vi "Autonomous Independent.vi"() -> ()   [LabVIEW 2013]
doc: "This VI is called when autonomous begins, and will automatically be terminated when autonomous ends. You can carry out timed or sensor driven robot movement independently without needing to return to the caller."
uses:
  <vilib>/Rock Robotics/WPI/Solenoid/WPI_SolenoidValue.ctl
  <vilib>/Rock Robotics/WPI/Relay/WPI_RelayValue.ctl
  Robot Global Data.vi
  <vilib>/Rock Robotics/WPI/Solenoid/WPI_SolenoidSetEnum.vi
  <vilib>/Rock Robotics/WPI/RobotDrive/WPI_RobotDriveArcadeDrive_Standard(NoSaturation).vi
  <vilib>/Rock Robotics/WPI/RobotDrive/WPI_RobotDriveGetSetRefNum.vi
  <vilib>/Rock Robotics/WPI/Joystick/WPI_JoystickGetSetRefNum.vi
  <vilib>/addons/control/pid/NI_PID_pid.lvlib
  <vilib>/addons/control/pid/pid.llb/PID (DBL).vi
  TargetType.ctl
panel:
  in  "Dist to drive":dbl=10000.0
  out "Go now or wait?":enum16{"Go Now", "Wait"}(ring)
  out "Stop Time":u32=1000
  in  "stop":bool
  out "Drive Forward Time":u32=1000
  out "Shoot Time":u32=1000
  out "Right? (T)":bool
  out "Position":T1
  in  "Launcher State":enum16{"Shoot", "Out", "Retract"}(ring)
  in  "Shooter Extended Time":u32=500
  out "Shooter Tick":u32
  out "Check Target Time":u32=5000
  out "Left?":bool
  out "Raise Arms Time":u32=1500
  in  "Up Position":dbl format="%.2f"
  out "Close Arms Time":u32=250
  out "Lower Arms Time":u32=1500
  in  "Down Position":dbl format="%.2f"
  out "Open Arms Time":u32=250
  in  "Auton State":T2(ring)
  out "Tick at start of Auton":u32
  out "Current Movement, for debugging":T3 {"Y Joystick Value" scale=1.0..-1.0; "X Joystick Value" scale=-1.0..1.0}
  in  "Array of robot movements":T4(array[cluster]) {"Y Joystick Value" scale=1.0..-1.0; "X Joystick Value" scale=-1.0..1.0}
  # "Be sure to right-click and choose Data Operations>>Make Current Value default if you want to save the array values with the VI"
  # "Main State Machine"
  # "Shooter State Machine"
  # "Disabled"
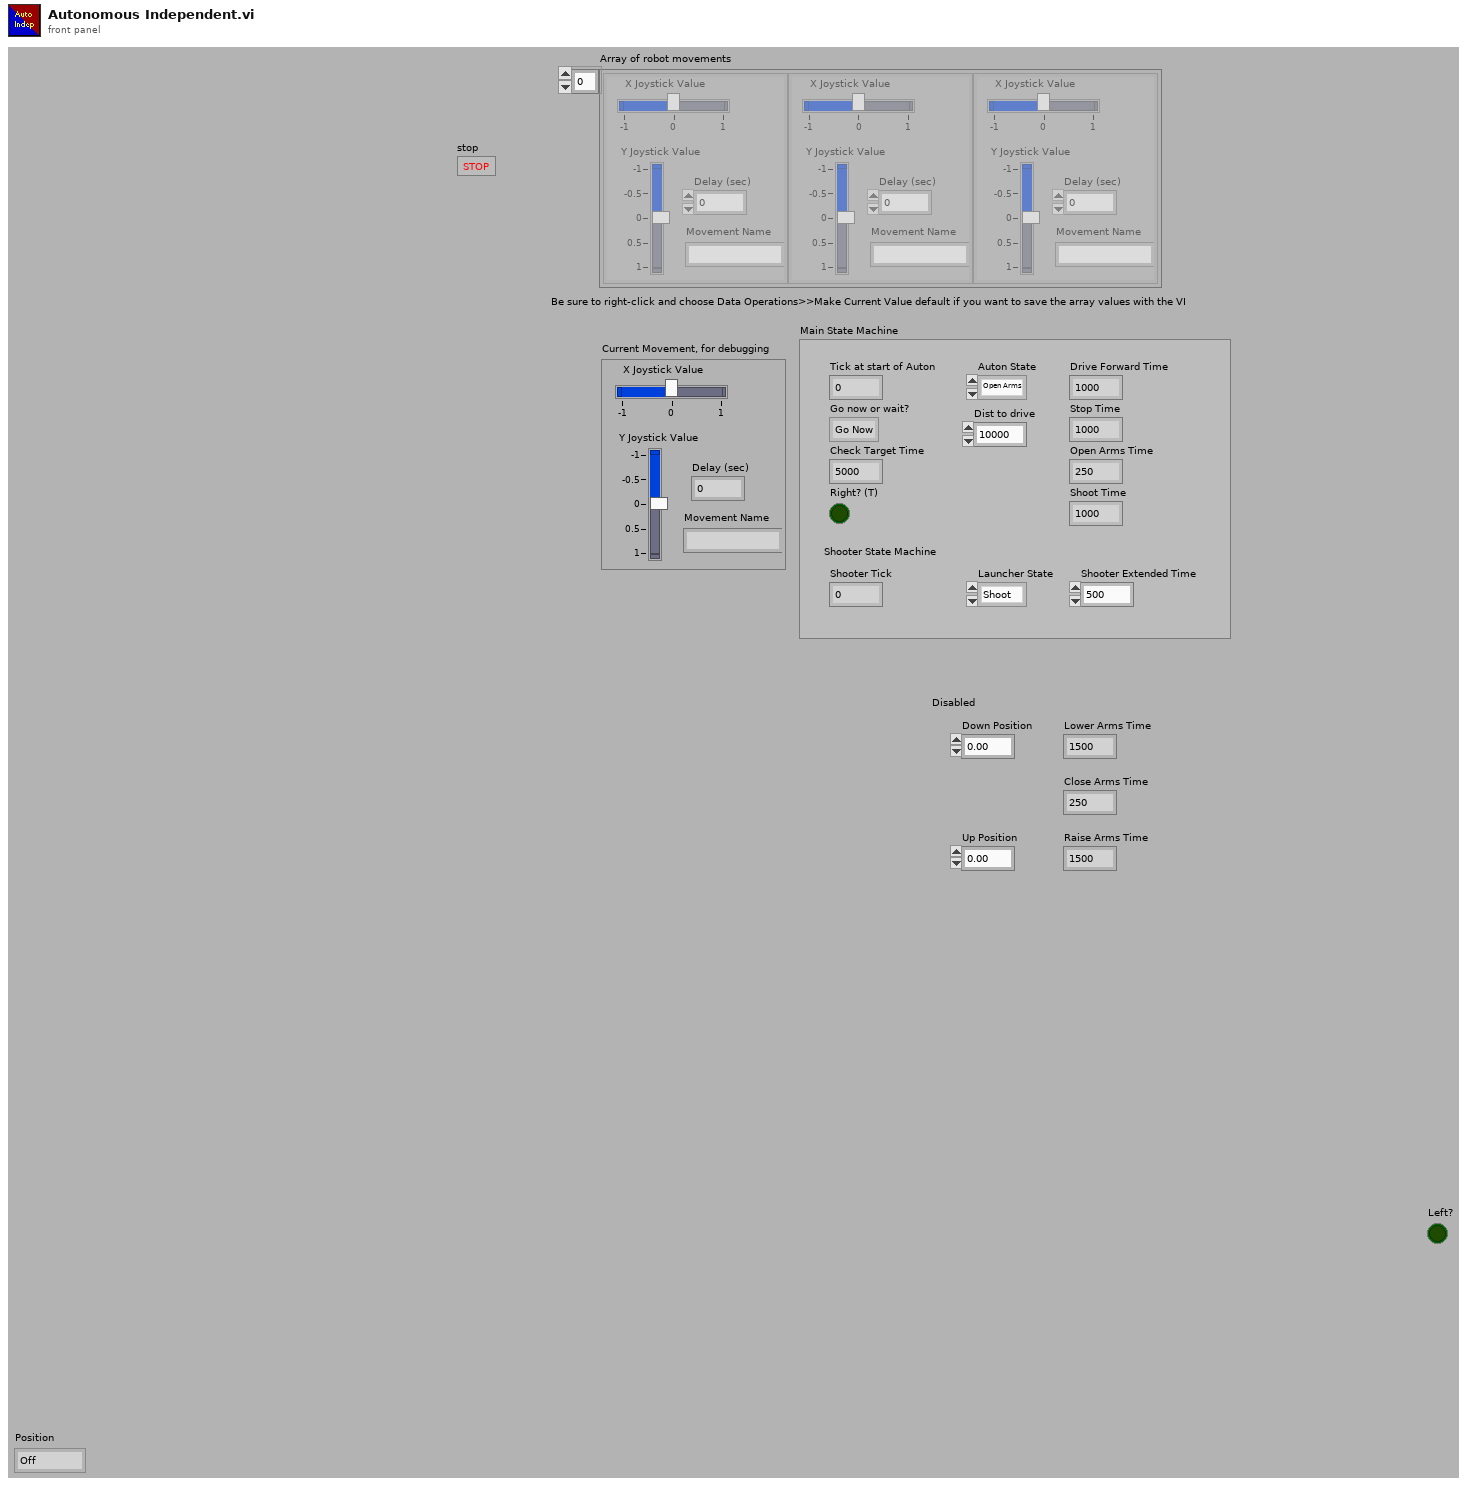
[diagram p1: front panel]
types:
  T1 = typedef "WPI_SolenoidValue.ctl" = enum16{"Off", "On", "Forward", "Reverse"}
  T2 = enum16{"Open Arms", "Lower Arms", "Close Arms", "Raise Arms", "Check Target", "Shoot", "Drive Forward", "Stop"}
  T3 = cluster{"X Joystick Value":dbl, "Y Joystick Value":dbl, "Delay (sec)":dbl, "Movement Name":string}
  T4 = cluster{"X Joystick Value":dbl, "Y Joystick Value":dbl, "Delay (sec)":dbl, "Movement Name":string}[]
  T5 = typedef "WPI_JoystickDevRef.ctl" = cluster{"Device":T6}
  T6 = typedef "WPI_JoystickDeviceEnum.ctl" = enum16{"USB 1", "USB 2", "USB 3", "USB 4", "Kinect 1", "Kinect 2"}
  T7 = cluster{"axis 1 (x)":dbl, "axis 2 (y)":dbl, "axis 3 (throttle)":dbl, "axis 4":dbl, "axis 5":dbl, "axis 6":dbl}
  T8 = typedef "WPI_RelayValue.ctl" = enum16{"Off", "On", "Forward", "Reverse"}
  T9 = typedef "TargetType.ctl" = enum16{"Not Hot", "Hot"}
  T10 = enum16{"Open Arms", "Lower Arms", "Close Arms", "Raise Arms", "Check Target", "Shoot", "Drive Forward"}
  T11 = cluster{"proportional gain (Kc)":dbl, "integral time (Ti, min)":dbl, "derivative time (Td, min)":dbl}
  T12 = typedef "WPI_SolenoidDevRef.ctl" = cluster{"DevStatus":errorcluster, "Solenoid Module":T13, "Forward Solenoid Channel":T14, "Reverse Solenoid Channel":T14}
  T13 = typedef "FPGA_TypedefSolenoidModule.ctl" = enum16{"Solenoid Module 1", "Solenoid Module 2"}
  T14 = typedef "WPI_SolenoidChannel.ctl" = enum8{"Solenoid 1", "Solenoid 2", "Solenoid 3", "Solenoid 4", "Solenoid 5", "Solenoid 6", "Solenoid 7", "Solenoid 8", "Invalid"}
  T15 = typedef "WPI_RelayDevRef.ctl" = cluster{"DevStatus":errorcluster, "Relay Channel":T16, "Digital Module":T17, "Relay Direction":T18}
  T16 = typedef "FPGA_DIORelayChannel.ctl" = enum8{"Relay 1", "Relay 2", "Relay 3", "Relay 4", "Relay 5", "Relay 6", "Relay 7", "Relay 8", "Invalid"}
  T17 = typedef "FPGA_TypedefDigitalModule.ctl" = enum16{"Digital Module 1", "Digital Module 2"}
  T18 = typedef "WPI_RelayDirection.ctl" = enum16{"Both directions", "Forward only", "Reverse only"}
  T19 = cluster{"Distance (ft)":dbl, "Target Center (-1 to 1)":cluster{"X":dbl, "Y":dbl}, "Left":bool, "State":T9}
  T20 = typedef "WPI_RobotDriveDevRef.ctl" = cluster{"DevStatus":errorcluster, "Motors[]":T21[], "Square Inputs":bool, "Max Output":dbl, "Isochronous":bool}
  T21 = typedef "WPI_MotorControlDeviceRef.ctl" = cluster{"DeviceStatus":errorcluster, "Type":enum16{"PWM", "CAN"}, "PWM":cluster{"Digital Module":T17, "PWM Channel":T22, "DeadBand":T23}, "CAN":cluster{"Device Number":u8, "Control Mode":T24, "Semaphore":T25, "Max Vout":dbl}, "Invert":bool, "TransformRef":T26, "InvTransformRef":T26}
  T22 = typedef "FPGA_DIOPWMChannel.ctl" = enum8{"PWM 1", "PWM 2", "PWM 3", "PWM 4", "PWM 5", "PWM 6", "PWM 7", "PWM 8", "PWM 9", "PWM 10", "Invalid"}
  T23 = typedef "WPI_PWMDeadband.ctl" = cluster{"Name":string, "maxPositivePwm":i32, "minPositivePwm":i32, "centerPwm":i32, "maxNegativePwm":i32, "minNegativePwm":i32, "angularRange":u16}
  T24 = typedef "WPI_CANJaguar_ControlMode.ctl" = enum8{"Percent VBus", "Current", "Speed", "Position", "Voltage"}
  T25 = typedef "Semaphore RefNum" = refnum<k1>
  T26 = typedef "WPI_PWMTransform_ConPane.ctl" = refnum<vi>
  T27 = typedef "WPI_AnalogChannelDevRef.ctl" = cluster{"DevStatus":errorcluster, "Analog Module":T28, "Analog Channel":T29}
  T28 = typedef "FPGA_TypedefAnalogModule.ctl" = enum16{"Analog Module 1", "Analog Module 2"}
  T29 = typedef "FPGA_AIChannel.ctl" = enum8{"AI 1", "AI 2", "AI 3", "AI 4", "AI 5", "AI 6", "AI 7", "AI 8", "Invalid"}
  T30 = typedef "WPI_EncoderDevRef.ctl" = cluster{"DevStatus":errorcluster, "EncoderIndex":T31, "CounterIndex":T32, "DistancePerCount":dbl, "Decoding Type":T33}
  T31 = typedef "FPGA_EncoderIdx.ctl" = enum8{"Enc 0", "Enc 1", "Enc 2", "Enc 3", "Invalid"}
  T32 = typedef "FPGA_CounterCtrSystemIndex.ctl" = enum8{"Ctr 0", "Ctr 1", "Ctr 2", "Ctr 3", "Ctr 4", "Ctr 5", "Ctr 6", "Ctr 7", "Invalid"}
  T33 = typedef "WPI_EncoderType.ctl" = enum16{"1x", "2x", "4x"}
  T34 = enum16{"Target Right", "No Target", "Target Left"}
  T35 = typedef "WPI_DigitalInputDevRef.ctl" = cluster{"DevStatus":errorcluster, "DIO Channel":T36, "Digital Module":T17}
  T36 = typedef "FPGA_DIOChannel.ctl" = enum8{"DIO 1", "DIO 2", "DIO 3", "DIO 4", "DIO 5", "DIO 6", "DIO 7", "DIO 8", "DIO 9", "DIO 10", "DIO 11", "DIO 12", "DIO 13", "DIO 14", "Invalid"}
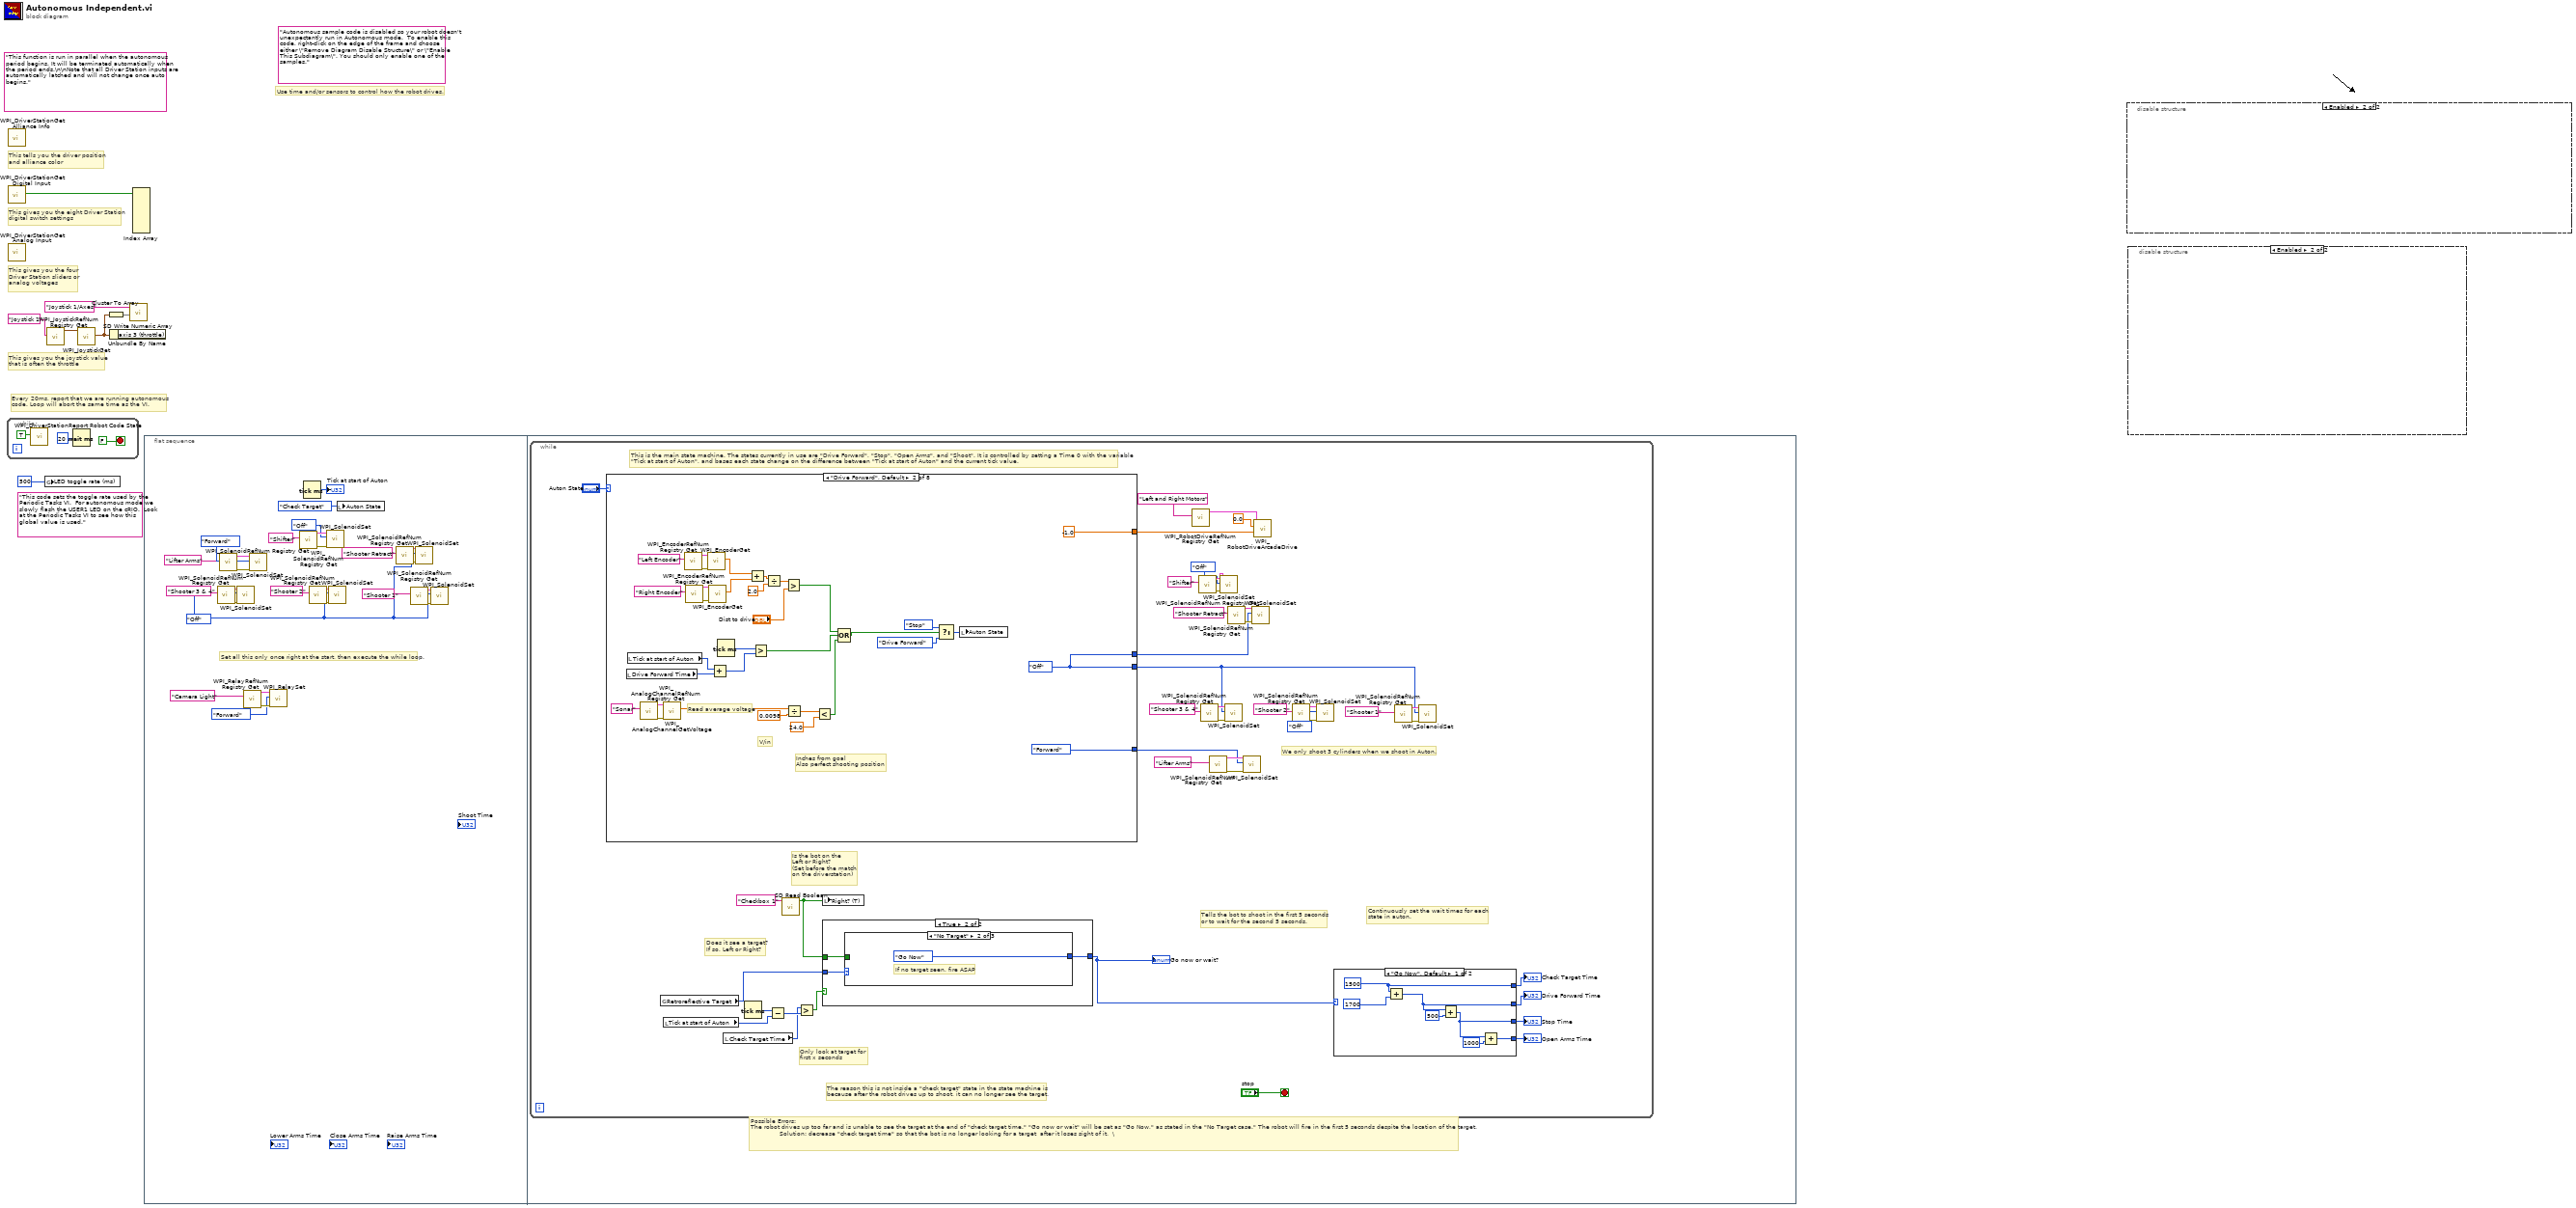
[diagram p0: block diagram]
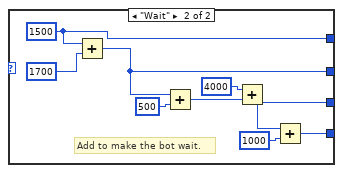
[diagram p2: hidden frame]
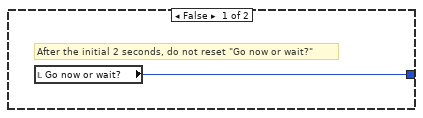
[diagram p3: hidden frame]
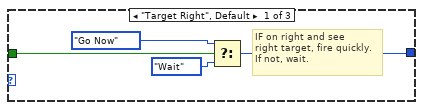
[diagram p4: hidden frame]
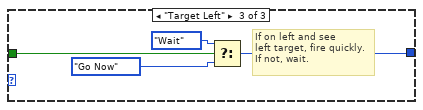
[diagram p5: hidden frame]
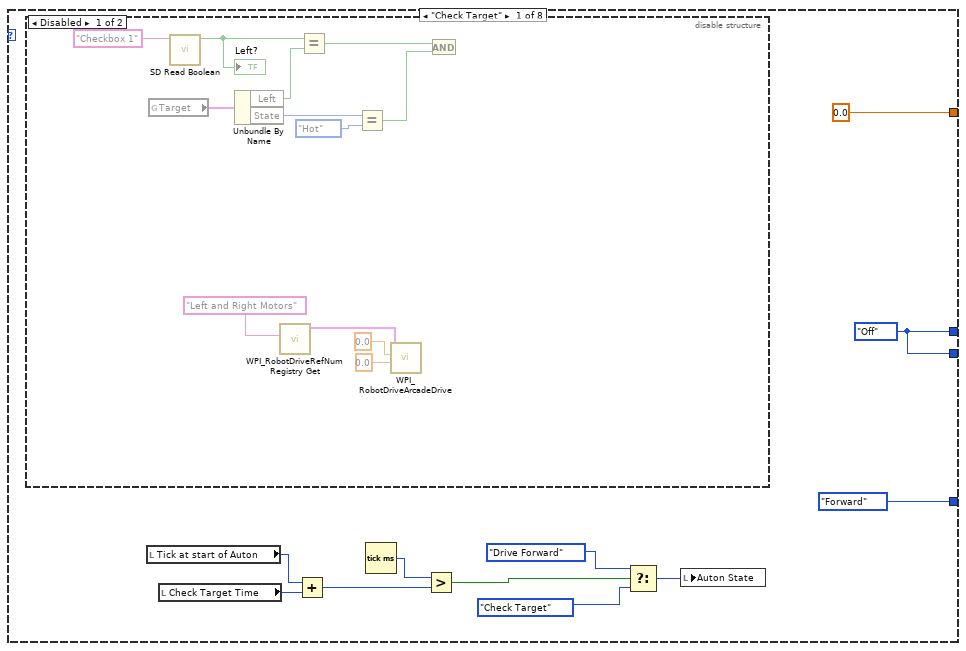
[diagram p6: hidden frame]
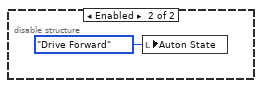
[diagram p7: hidden frame]
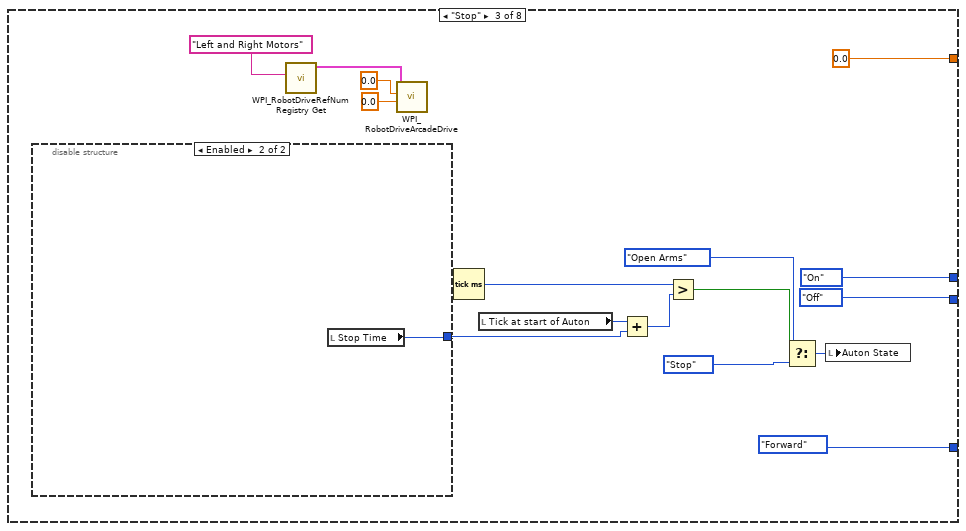
[diagram p8: hidden frame]
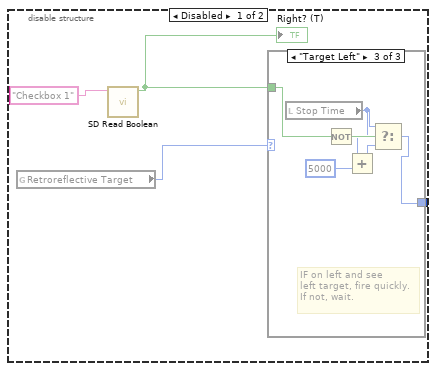
[diagram p9: hidden frame]
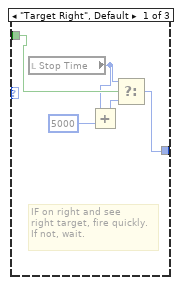
[diagram p10: hidden frame]
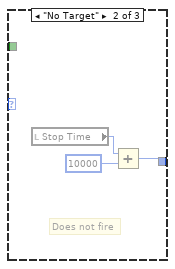
[diagram p11: hidden frame]
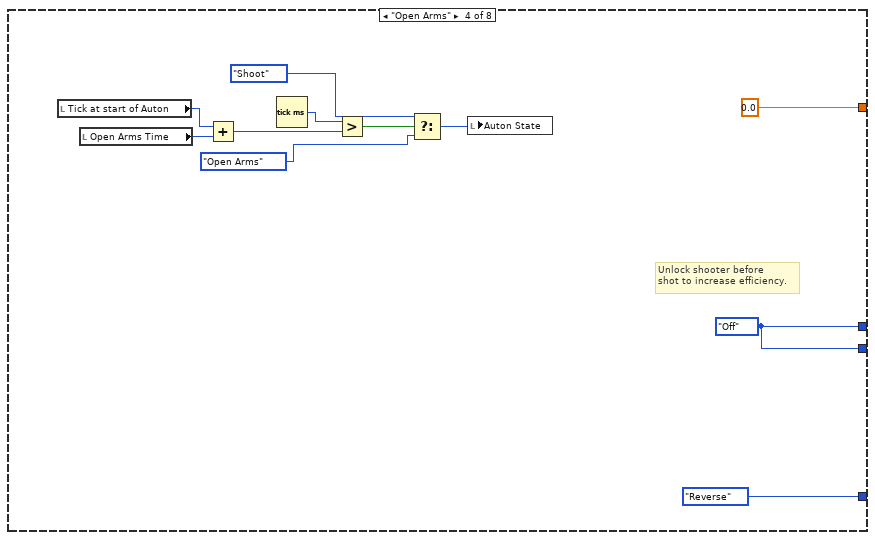
[diagram p12: hidden frame]
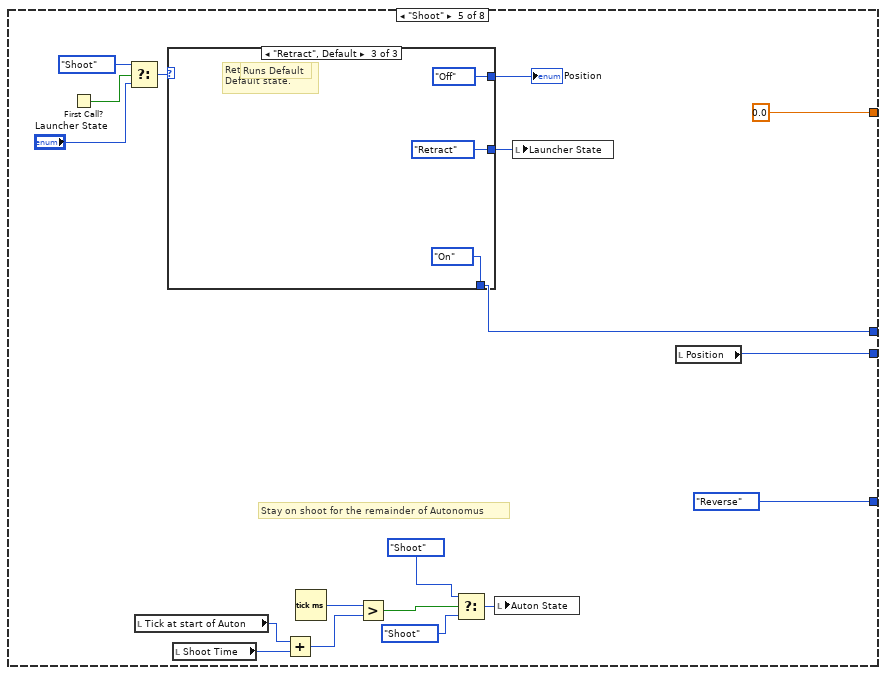
[diagram p13: hidden frame]
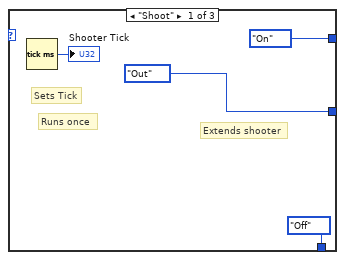
[diagram p14: hidden frame]
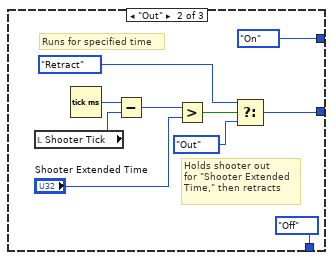
[diagram p15: hidden frame]
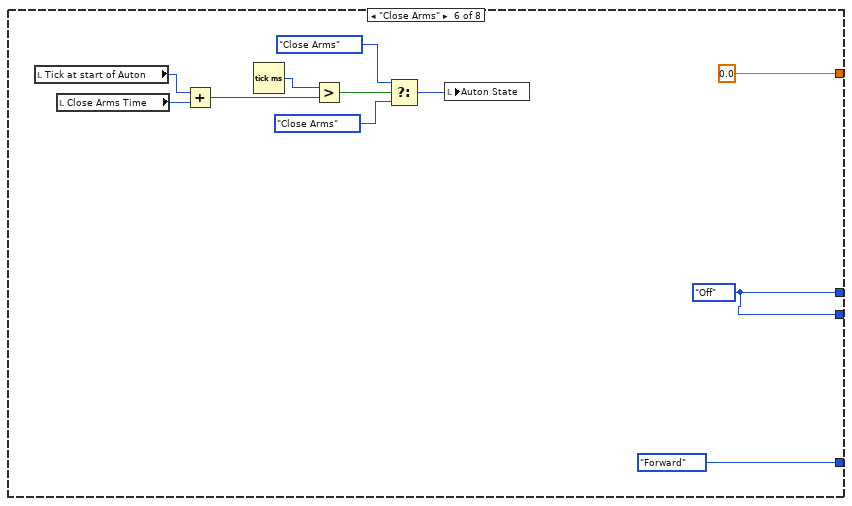
[diagram p16: hidden frame]
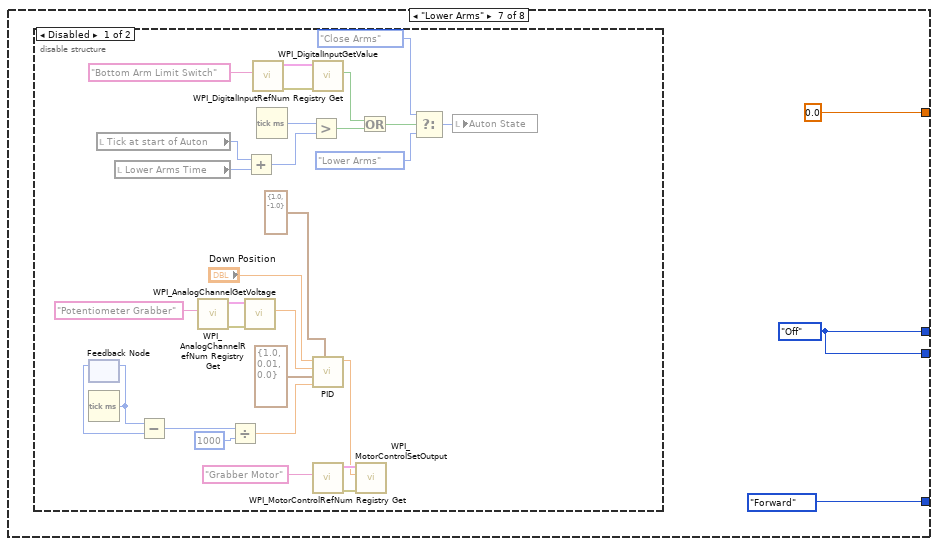
[diagram p17: hidden frame]
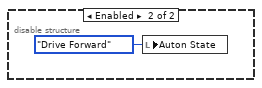
[diagram p18: hidden frame]
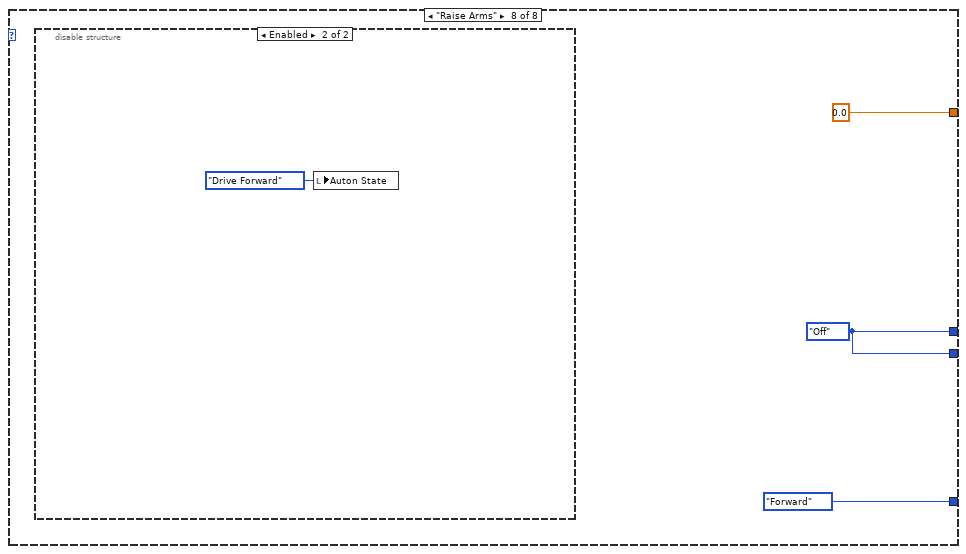
[diagram p19: hidden frame]
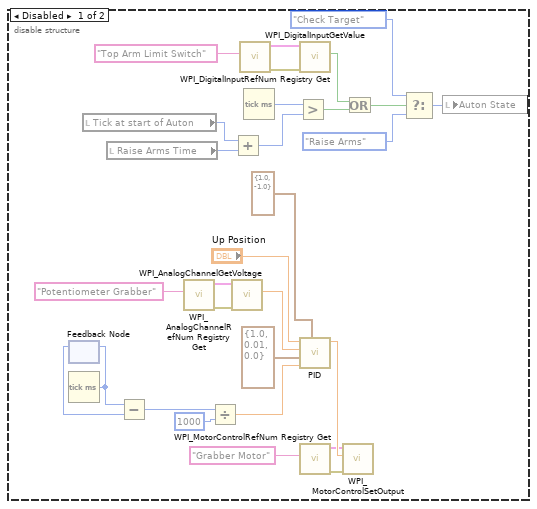
[diagram p20: hidden frame]
diagram:
  (unwired) "This code sets the toggle rate used by the Periodic Tasks VI.  For autonomous mode we slowly flash the USER1 LED on the cRIO.  Look at the Periodic Tasks VI to see how this global value is used."
  (unwired) "Autonomous sample code is disabled so your robot doesn't unexpectantly run in Autonomous mode.  To enable this code, right-click on the edge of the frame and choose either \"Remove Diagram Disable Structure\" or \"Enable This Subdiagram\". You should only enable one of the samples."
  (unwired) "This function is run in parallel when the autonomous period begins. It will be terminated automatically when the period ends.\n\nNote that all Driver Station inputs are automatically latched and will not change once auto begins."
  # "Every 20ms, report that we are running autonomous\ncode. Loop will abort the same time as the VI."
  # "This gives you the joystick value\nthat is often the throttle"
  # "Use time and/or sensors to control how the robot drives."
  # "This tells you the driver position\nand alliance color"
  # "This gives you the eight Driver Station\ndigital switch settings"
  # "This gives you the four\nDriver Station sliders or\nanalog voltages"
  n1 = while {
    stop <- FALSE stop-if-true
    n2 = call <vilib>:"WPI_DriverStationReport Robot Code State.vi"("Autonomous"=TRUE) -> ()  [unwired: 10 in, 1 out]
    n3 = Wait (ms)(milliseconds to wait=u32 20) -> ()  [unwired: 1 out]
  }
  n4 = call <vilib>:"WPI_DriverStationGet Alliance Info.vi"() -> ()  [unwired: 12 out]
  n5 = call <vilib>:"WPI_DriverStationGet Digital Input.vi"() -> ("Driver Station Digital Input (1-8)"=w7:bool[])  [unwired: 11 out]
  n6 = call <vilib>:"WPI_DriverStationGet Analog Input.vi"() -> ()  [unwired: 12 out]
  n7 = global write "Robot Global Data.vi" "LED toggle rate (ms)"(u32 500 ("LED ms toggle rate")) -> ()
  n8 = call <vilib>:"WPI_JoystickRefNum Registry Get.vi"("refnum name"="Joystick 1") -> ("JoystickDevRef"=w5:T5)  [unwired: 1 in, 9 out]
  n9 = call <vilib>:"WPI_JoystickGet.vi"("JoystickDevRef"=w5) -> ("Axes"=w2:T7)  [unwired: 1 in, 5 out]
  n10 = Cluster To Array(cluster=w2) -> (array=w3:dbl[])
  n11 = Unbundle By Name(w2) -> ()  [unwired: 1 out]
  n12 = call <vilib>:"SD Write Numeric Array.vi"("Numeric Array"=w3, "Name"="Joystick 1/Axes") -> ()  [unwired: 8 in, 2 out]
  n13 = Index Array(array=w7) -> ()  [unwired: 8 in, 8 out]
  n14 = flat-sequence {
    frame #0 {
      w23 = WPI_SolenoidValue."Off" ("x")
      # "Set all this only once right at the start, then execute the while loop."
      n15 = call <vilib>:"WPI_SolenoidRefNum Registry Get.vi"("refnum name"="Shooter 3 & 4") -> ("error out"=w30:errorcluster, "SolenoidDevRef"=w34:T12)  [unwired: 9 in]
      n16 = call <vilib>:"WPI_SolenoidRefNum Registry Get.vi"("refnum name"="Lifter Arms") -> ("error out"=w17:errorcluster, "SolenoidDevRef"=w18:T12)  [unwired: 9 in]
      n17 = call-poly <vilib>:"WPI_SolenoidSet.vi"("error in (no error)"=w30, "Value"=w23, "SolenoidDevRef"=w34) -> ()  [unwired: 7 in, 2 out]
      n18 = call <vilib>:"WPI_RelayRefNum Registry Get.vi"("refnum name"="Camera Light") -> ("error out"=w14:errorcluster, "RelayDevRef"=w13:T15)  [unwired: 9 in]
      n19 = call-poly <vilib>:"WPI_SolenoidSet.vi"("error in (no error)"=w17, "Value"=WPI_SolenoidValue."Forward", "SolenoidDevRef"=w18) -> ()  [unwired: 7 in, 2 out]
      n20 = call <vilib>:"WPI_RelaySet.vi"("error in (no error)"=w14, "RelayValue"=WPI_RelayValue."Forward", "RelayDevRef"=w13) -> ()  [unwired: 7 in, 2 out]
      n21 = call <vilib>:"WPI_SolenoidRefNum Registry Get.vi"("refnum name"="Shifter") -> ("error out"=w21:errorcluster, "SolenoidDevRef"=w20:T12)  [unwired: 9 in]
      n22 = Tick Count (ms)() -> (millisecond timer value=→"Tick at start of Auton":u32)
      n23 = call <vilib>:"WPI_SolenoidRefNum Registry Get.vi"("refnum name"="Shooter 2") -> ("error out"=w27:errorcluster, "SolenoidDevRef"=w35:T12)  [unwired: 9 in]
      n24 = call-poly <vilib>:"WPI_SolenoidSet.vi"("error in (no error)"=w21, "Value"=WPI_SolenoidValue."Off", "SolenoidDevRef"=w20) -> ()  [unwired: 7 in, 2 out]
      n25 = call-poly <vilib>:"WPI_SolenoidSet.vi"("error in (no error)"=w27, "Value"=w23, "SolenoidDevRef"=w35) -> ()  [unwired: 7 in, 2 out]
      n26 = local write "Auton State"(T2."Check Target" ("Auton State")) -> ()
      n27 = call <vilib>:"WPI_SolenoidRefNum Registry Get.vi"("refnum name"="Shooter Retract") -> ("error out"=w25:errorcluster, "SolenoidDevRef"=w24:T12)  [unwired: 9 in]
      n28 = call <vilib>:"WPI_SolenoidRefNum Registry Get.vi"("refnum name"="Shooter 1") -> ("error out"=w32:errorcluster, "SolenoidDevRef"=w33:T12)  [unwired: 9 in]
      n29 = call-poly <vilib>:"WPI_SolenoidSet.vi"("error in (no error)"=w25, "Value"=w23, "SolenoidDevRef"=w24) -> ()  [unwired: 7 in, 2 out]
      n30 = call-poly <vilib>:"WPI_SolenoidSet.vi"("error in (no error)"=w32, "Value"=w23, "SolenoidDevRef"=w33) -> ()  [unwired: 7 in, 2 out]
    }
    frame #1 {
      # "Possible Errors:\nThe robot drives up too far and is unable to see the target at the end of \"check target time.\" \"Go now or wait\" will be set as \"Go Now,\" as stated in the \"No Target case.\" The robot will fire in the first 5 seconds despite the location of the target.\n               Solution: decrease \"check target time\" so that the bot is no longer looking for a target  after it loses sight of it.  \\"
      n31 = while {
        stop <- "stop" stop-if-true
        # "We only shoot 3 cylinders when we shoot in Auton."
        # "This is the main state machine. The states currently in use are \"Drive Forward\", \"Stop\", \"Open Arms\", and \"Shoot\". It is controlled by setting a Time 0 with the variable\n\"Tick at start of Auton\", and bases each state change on the difference between \"Tick at start of Auton\" and the current tick value."
        # "The reason this is not inside a \"check target\" state in the state machine is \nbecause after the robot drives up to shoot, it can no longer see the target."
        # "Continuously set the wait times for each\nstate in auton."
        # "Tells the bot to shoot in the first 5 seconds\nor to wait for the second 5 seconds."
        # "Is the bot on the\nLeft or Right?\n(Set before the match\non the driverstation)"
        # "Does it see a target?\nIf so, Left or Right?"
        # "Only look at target for \nfirst x seconds"
        n32 = case shown="\"Drive Forward\", Default" "Auton State" {
          tunnel: [w117 w159 WPI_SolenoidValue."Off" ("x") w204 w216 w252 w261 w294] -> w65
          tunnel: [w117 w159 WPI_SolenoidValue."On" ("x") w204 w213 w252 w261 w294] -> w64
          tunnel: [0.0 ("Y axis value") -1.0 ("Y axis value") 0.0 ("Y axis value") 0.0 ("Y axis value") 0.0 ("Y axis value") 0.0 ("Y axis value") 0.0 ("Y axis value") 0.0 ("Y axis value")] -> w60
          tunnel: [WPI_SolenoidValue."Forward" ("Value") WPI_SolenoidValue."Forward" ("Value") WPI_SolenoidValue."Forward" ("Value") WPI_SolenoidValue."Reverse" ("Value") WPI_SolenoidValue."Reverse" ("Value") WPI_SolenoidValue."Forward" ("Value") WPI_SolenoidValue."Forward" ("Value") WPI_SolenoidValue."Forward" ("Value")] -> w52
          frame "Check Target" {
            w117 = WPI_SolenoidValue."Off" ("x")
            n33 = disable-structure shown="Disabled" {
              frame Disabled {
                n34 = global read "Robot Global Data.vi" "Target"() -> (w132:T19)
                n35 = call <vilib>:"SD Read Boolean.vi"("Name"="Checkbox 1" ("refnum name")) -> ("Boolean"=w127:bool)  [unwired: 8 in, 2 out]
                "Left?" <- w127
                n36 = Unbundle By Name(w132) -> ("Left"=w128:bool, "State"=w131:T9)
                n37 = call <vilib>:"WPI_RobotDriveRefNum Registry Get.vi"("refnum name"="Left and Right Motors") -> ("RobotDriveDevRef"=w120:T20)  [unwired: 1 in, 9 out]
                n38 = Equal?(x=w127, y=w128) -> (x = y?=w125:bool)
                n39 = Equal?(x=w131, y=TargetType."Hot") -> (x = y?=w126:bool)
                n40 = call-poly <vilib>:"WPI_RobotDriveArcadeDrive.vi"("Y axis value"=0.0, "X axis value"=0.0, "RobotDriveDevRef"=w120) -> ()  [unwired: 6 in, 3 out]
                n41 = And(x=w125, y=w126) -> (x .and. y?=w124:bool)
              }
              frame Enabled {
                n42 = local write "Auton State"(T2."Drive Forward" ("Auton State")) -> ()
              }
            }
            n43 = local read "Tick at start of Auton"() -> (w113:u32)
            n44 = local read "Check Target Time"() -> (w111:u32)
            n45 = Add(x=w113, y=w111) -> (x+y=w112:u32)
            n46 = Tick Count (ms)() -> (millisecond timer value=w114:u32)
            n47 = Greater?(x=w114, y=w112) -> (0:w109:bool)
            n48 = Select(t=T2."Drive Forward" ("Auton State"), s=w109, f=T2."Check Target" ("Auton State")) -> (s? t:f=w115:T2)
            n49 = local write "Auton State"(w115) -> ()
          }
          frame "Drive Forward", Default {
            w159 = WPI_SolenoidValue."Off" ("Value")
            # "Inches from goal\nAlso perfect shooting position"
            # "V/in"
            # "Read average voltage"
            n50 = local read "Drive Forward Time"() -> (w166:u32)
            n51 = local read "Tick at start of Auton"() -> (w164:u32)
            n52 = call <vilib>:"WPI_AnalogChannelRefNum Registry Get.vi"("refnum name"="Sonar") -> ("error out"=w143:errorcluster, "AIDeviceRef"=w138:T27)  [unwired: 9 in]
            n53 = call <vilib>:"WPI_AnalogChannelGetVoltage.vi"("error in (no error)"=w143, "AIDeviceRef"=w138) -> ("Voltage"=w144:dbl)  [unwired: 7 in, 2 out]
            n54 = call <vilib>:"WPI_EncoderRefNum Registry Get.vi"("refnum name"="Left Encoder") -> ("error out"=w156:errorcluster, "EncoderDevRef"=w155:T30)  [unwired: 9 in]
            n55 = call <vilib>:"WPI_EncoderRefNum Registry Get.vi"("refnum name"="Right Encoder") -> ("error out"=w151:errorcluster, "EncoderDevRef"=w152:T30)  [unwired: 9 in]
            n56 = call <vilib>:"WPI_EncoderGet.vi"("error in (no error)"=w156, "EncoderDevRef"=w155) -> ("Distance"=w150:dbl)  [unwired: 4 in, 5 out]
            n57 = call <vilib>:"WPI_EncoderGet.vi"("error in (no error)"=w151, "EncoderDevRef"=w152) -> ("Distance"=w149:dbl)  [unwired: 4 in, 5 out]
            n58 = Add(x=w164, y=w166) -> (x+y=w165:u32)
            n59 = Tick Count (ms)() -> (millisecond timer value=w163:u32)
            n60 = Add(x=w150, y=w149) -> (x+y=w148:dbl)
            n61 = Greater?(x=w163, y=w165) -> (0:w135:bool)
            n62 = Divide(x=w148, y=2.0) -> (x/y=w146:dbl)
            n63 = Greater?(x=w146, y="Dist to drive") -> (0:w136:bool)
            n64 = Divide(x=w144, y=0.0098) -> (x/y=w140:dbl)
            n65 = Less?(x=w140, y=24.0) -> (x < y?=w134:bool)
            n66 = Compound Arithmetic op=OR(w136, w135, w134) -> (w137:bool)
            n67 = Select(t=T2."Stop" ("Auton State"), s=w137, f=T2."Drive Forward" ("Auton State")) -> (s? t:f=w162:T2)
            n68 = local write "Auton State"(w162) -> ()
          }
          frame "Stop" {
            n69 = disable-structure shown="Enabled" {
              disable-tunnel: [w183 w201] -> w167
              frame Disabled {
                n70 = global read "Robot Global Data.vi" "Retroreflective Target"() -> (w185:T34)
                n71 = call <vilib>:"SD Read Boolean.vi"("Name"="Checkbox 1" ("refnum name")) -> ("Boolean"=w184:bool)  [unwired: 8 in, 2 out]
                "Right? (T)" <- w184
                n72 = case shown="\"Target Left\"" w185 {
                  tunnel: w184 -> [w188 _ w200]
                  tunnel: [w189 w194 w195] -> w183
                  frame "Target Right", Default {
                    # "IF on right and see\nright target, fire quickly.\nIf not, wait."
                    n73 = local read "Stop Time"() -> (w187:u32)
                    n74 = Add(x=w187, y=u32 5000) -> (x+y=w191:u32)
                    n75 = Select(t=w187, s=w188, f=w191) -> (s? t:f=w189:u32)
                  }
                  frame "No Target" {
                    # "Does not fire"
                    n76 = local read "Stop Time"() -> (w193:u32)
                    n77 = Add(x=w193, y=u32 10000) -> (x+y=w194:u32)
                  }
                  frame "Target Left" {
                    # "IF on left and see\nleft target, fire quickly.\nIf not, wait."
                    n78 = local read "Stop Time"() -> (w198:u32)
                    n79 = Not(x=w200) -> (.not. x?=w199:bool)
                    n80 = Add(x=w198, y=u32 5000) -> (x+y=w197:u32)
                    n81 = Select(t=w198, s=w199, f=w197) -> (s? t:f=w195:u32)
                  }
                }
              }
              frame Enabled {
                n82 = local read "Stop Time"() -> (w201:u32)
              }
            }
            n83 = call <vilib>:"WPI_RobotDriveRefNum Registry Get.vi"("refnum name"="Left and Right Motors") -> ("RobotDriveDevRef"=w179:T20)  [unwired: 1 in, 9 out]
            n84 = call-poly <vilib>:"WPI_RobotDriveArcadeDrive.vi"("Y axis value"=0.0, "X axis value"=0.0, "RobotDriveDevRef"=w179) -> ()  [unwired: 6 in, 3 out]
            n85 = Tick Count (ms)() -> (millisecond timer value=w173:u32)
            n86 = local read "Tick at start of Auton"() -> (w174:u32)
            n87 = Add(x=w174, y=w167) -> (x+y=w175:u32)
            n88 = Greater?(x=w173, y=w175) -> (0:w171:bool)
            n89 = Select(t=T2."Open Arms" ("Auton State"), s=w171, f=T2."Stop" ("Auton State")) -> (s? t:f=w172:T2)
            n90 = local write "Auton State"(w172) -> ()
          }
          frame "Open Arms" {
            w204 = WPI_SolenoidValue."Off" ("Value")
            # "Unlock shooter before\nshot to increase efficiency."
            n91 = local read "Tick at start of Auton"() -> (w211:u32)
            n92 = local read "Open Arms Time"() -> (w208:u32)
            n93 = Add(x=w211, y=w208) -> (x+y=w210:u32)
            n94 = Tick Count (ms)() -> (millisecond timer value=w212:u32)
            n95 = Greater?(x=w212, y=w210) -> (0:w209:bool)
            n96 = Select(t=T2."Shoot" ("Auton State"), s=w209, f=T2."Open Arms" ("Auton State")) -> (s? t:f=w205:T2)
            n97 = local write "Auton State"(w205) -> ()
          }
          frame "Shoot" {
            # "Stay on shoot for the remainder of Autonomus"
            n98 = First Call?() -> (First Call?: T/F=w225:bool)
            n99 = Select(t=enum16{"Shoot", "Out", "Retract"}."Shoot", s=w225, f="Launcher State") -> (s? t:f=w229:enum16{"Shoot", "Out", "Retract"})
            n100 = local read "Tick at start of Auton"() -> (w222:u32)
            n101 = case shown="\"Retract\", Default" w229 {
              tunnel: [WPI_SolenoidValue."On" ("Value") WPI_SolenoidValue."On" ("Value") WPI_SolenoidValue."Off" ("Value")] -> w226
              tunnel: [enum16{"Shoot", "Out", "Retract"}."Out" ("Launcher State") w237 enum16{"Shoot", "Out", "Retract"}."Retract" ("Launcher State")] -> w227
              tunnel: [WPI_SolenoidValue."Off" ("t") WPI_SolenoidValue."Off" ("t") WPI_SolenoidValue."On" ("t")] -> w213
              frame "Shoot" {
                # "Runs once"
                # "Sets Tick"
                # "Extends shooter"
                n102 = Tick Count (ms)() -> (millisecond timer value=→"Shooter Tick":u32)
              }
              frame "Out" {
                # "Runs for specified time"
                # "Holds shooter out\nfor \"Shooter Extended\nTime,\" then retracts"
                n103 = local read "Shooter Tick"() -> (w243:u32)
                n104 = Tick Count (ms)() -> (millisecond timer value=w244:u32)
                n105 = Subtract(x=w244, y=w243) -> (x-y=w242:u32)
                n106 = Greater?(x=w242, y="Shooter Extended Time") -> (0:w241:bool)
                n107 = Select(t=enum16{"Shoot", "Out", "Retract"}."Retract" ("Launcher State"), s=w241, f=enum16{"Shoot", "Out", "Retract"}."Out" ("Launcher State")) -> (s? t:f=w237:enum16{"Shoot", "Out", "Retract"})
              }
              frame "Retract", Default {
                # "Runs Default"
                # "Retracts Shooter, \nDefault state."
              }
            }
            "Position" <- w226
            n108 = local read "Shoot Time"() -> (w224:u32)
            n109 = Add(x=w222, y=w224) -> (x+y=w223:u32)
            n110 = Tick Count (ms)() -> (millisecond timer value=w221:u32)
            n111 = Greater?(x=w221, y=w223) -> (0:w219:bool)
            n112 = Select(t=T2."Shoot" ("Auton State"), s=w219, f=T2."Shoot" ("Auton State")) -> (s? t:f=w220:T2)
            n113 = local write "Auton State"(w220) -> ()
            n114 = local write "Launcher State"(w227) -> ()
            n115 = local read "Position"() -> (w216:T1)
          }
          frame "Close Arms" {
            w252 = WPI_SolenoidValue."Off" ("x")
            n116 = local read "Tick at start of Auton"() -> (w255:u32)
            n117 = local read "Close Arms Time"() -> (w258:u32)
            n118 = Add(x=w255, y=w258) -> (x+y=w256:u32)
            n119 = Tick Count (ms)() -> (millisecond timer value=w254:u32)
            n120 = Greater?(x=w254, y=w256) -> (0:w257:bool)
            n121 = Select(t=T2."Close Arms" ("Auton State"), s=w257, f=T2."Close Arms" ("Auton State")) -> (s? t:f=w253:T2)
            n122 = local write "Auton State"(w253) -> ()
          }
          frame "Lower Arms" {
            w261 = WPI_SolenoidValue."Off" ("x")
            n123 = disable-structure shown="Disabled" {
              frame Disabled {
                n124 = feedback #1() -> (w285:u32)  [unwired: 1 in]
                n125 = Tick Count (ms)() -> (millisecond timer value=w286:u32)
                n126 = feedback-in #1(w286) -> ()
                n127 = local read "Tick at start of Auton"() -> (w267:u32)
                n128 = local read "Lower Arms Time"() -> (w265:u32)
                n129 = Subtract(x=w286, y=w285) -> (x-y=w284:u32)
                n130 = call <vilib>:"WPI_AnalogChannelRefNum Registry Get.vi"("refnum name"="Potentiometer Grabber") -> ("error out"=w288:errorcluster, "AIDeviceRef"=w289:T27)  [unwired: 9 in]
                n131 = Divide(x=w284, y=u32 1000) -> (x/y=w282:dbl)
                n132 = call <vilib>:"WPI_AnalogChannelGetVoltage.vi"("error in (no error)"=w288, "AIDeviceRef"=w289) -> ("Voltage"=w276:dbl)  [unwired: 7 in, 2 out]
                n133 = Add(x=w267, y=w265) -> (x+y=w266:u32)
                n134 = call <vilib>:"WPI_DigitalInputRefNum Registry Get.vi"("refnum name"="Bottom Arm Limit Switch") -> ("error out"=w271:errorcluster, "DigitalInputDevRef"=w270:T35)  [unwired: 9 in]
                n135 = Tick Count (ms)() -> (millisecond timer value=w268:u32)
                n136 = Greater?(x=w268, y=w266) -> (0:w262:bool)
                n137 = call <vilib>:"WPI_DigitalInputGetValue.vi"("error in (no error)"=w271, "DigitalInputDevRef"=w270) -> ("Value"=w263:bool)  [unwired: 7 in, 2 out]
                n138 = call-poly <vilib>:"PID.vi"("output range"=cluster{"output high":dbl, "output low":dbl} {"output high"=1.0, "output low"=-1.0}, "dt (s)"=w282, "PID gains"=T11 {"proportional gain (Kc)"=1.0, "integral time (Ti, min)"=0.01, "derivative time (Td, min)"=0.0}, "process variable"=w276, "setpoint"="Down Position") -> ("output"=w279:dbl)  [unwired: 5 in, 1 out]
                n139 = call <vilib>:"WPI_MotorControlRefNum Registry Get.vi"("refnum name"="Grabber Motor") -> ("error out"=w281:errorcluster, "MotorControlDevRef"=w280:T21)  [unwired: 9 in]
                n140 = call <vilib>:"WPI_MotorControlSetOutput.vi"("error in (no error)"=w281, "Output"=w279, "MotorControlDevRef"=w280) -> ()  [unwired: 6 in, 3 out]
                n141 = Or(x=w263, y=w262) -> (x .or. y?=w264:bool)
                n142 = Select(t=T10."Close Arms", s=w264, f=T10."Lower Arms") -> (s? t:f=w274:T10)
                n143 = local write "Auton State"(w274) -> ()
              }
              frame Enabled {
                n144 = local write "Auton State"(T2."Drive Forward" ("Auton State")) -> ()
              }
            }
          }
          frame "Raise Arms" {
            w294 = WPI_SolenoidValue."Off" ("x")
            n145 = disable-structure shown="Enabled" {
              frame Disabled {
                n146 = feedback #2() -> (w300:u32)  [unwired: 1 in]
                n147 = Tick Count (ms)() -> (millisecond timer value=w299:u32)
                n148 = feedback-in #2(w299) -> ()
                n149 = local read "Tick at start of Auton"() -> (w318:u32)
                n150 = local read "Raise Arms Time"() -> (w320:u32)
                n151 = Subtract(x=w299, y=w300) -> (x-y=w301:u32)
                n152 = call <vilib>:"WPI_AnalogChannelRefNum Registry Get.vi"("refnum name"="Potentiometer Grabber") -> ("error out"=w297:errorcluster, "AIDeviceRef"=w296:T27)  [unwired: 9 in]
                n153 = Divide(x=w301, y=u32 1000) -> (x/y=w303:dbl)
                n154 = call <vilib>:"WPI_AnalogChannelGetVoltage.vi"("error in (no error)"=w297, "AIDeviceRef"=w296) -> ("Voltage"=w309:dbl)  [unwired: 7 in, 2 out]
                n155 = Add(x=w318, y=w320) -> (x+y=w319:u32)
                n156 = call <vilib>:"WPI_DigitalInputRefNum Registry Get.vi"("refnum name"="Top Arm Limit Switch") -> ("error out"=w314:errorcluster, "DigitalInputDevRef"=w315:T35)  [unwired: 9 in]
                n157 = Tick Count (ms)() -> (millisecond timer value=w317:u32)
                n158 = Greater?(x=w317, y=w319) -> (0:w323:bool)
                n159 = call <vilib>:"WPI_DigitalInputGetValue.vi"("error in (no error)"=w314, "DigitalInputDevRef"=w315) -> ("Value"=w322:bool)  [unwired: 7 in, 2 out]
                n160 = call-poly <vilib>:"PID.vi"("output range"=cluster{"output high":dbl, "output low":dbl} {"output high"=1.0, "output low"=-1.0}, "dt (s)"=w303, "PID gains"=T11 {"proportional gain (Kc)"=1.0, "integral time (Ti, min)"=0.01, "derivative time (Td, min)"=0.0}, "process variable"=w309, "setpoint"="Up Position") -> ("output"=w306:dbl)  [unwired: 5 in, 1 out]
                n161 = call <vilib>:"WPI_MotorControlRefNum Registry Get.vi"("refnum name"="Grabber Motor") -> ("error out"=w304:errorcluster, "MotorControlDevRef"=w305:T21)  [unwired: 9 in]
                n162 = call <vilib>:"WPI_MotorControlSetOutput.vi"("error in (no error)"=w304, "Output"=w306, "MotorControlDevRef"=w305) -> ()  [unwired: 6 in, 3 out]
                n163 = Or(x=w322, y=w323) -> (x .or. y?=w321:bool)
                n164 = Select(t=T10."Check Target", s=w321, f=T10."Raise Arms") -> (s? t:f=w311:T10)
                n165 = local write "Auton State"(w311) -> ()
              }
              frame Enabled {
                n166 = local write "Auton State"(T2."Drive Forward" ("Auton State")) -> ()
              }
            }
          }
        }
        n167 = global read "Robot Global Data.vi" "Retroreflective Target"() -> (w48:T34)
        n168 = local read "Tick at start of Auton"() -> (w46:u32)
        n169 = local read "Check Target Time"() -> (w39:u32)
        n170 = Tick Count (ms)() -> (millisecond timer value=w47:u32)
        n171 = Subtract(x=w47, y=w46) -> (x-y=w45:u32)
        n172 = call <vilib>:"SD Read Boolean.vi"("Name"="Checkbox 1" ("refnum name")) -> ("Boolean"=w49:bool)  [unwired: 8 in, 2 out]
        n173 = Greater?(x=w39, y=w45) -> (0:w44:bool)
        n174 = local write "Right? (T)"(w49) -> ()
        n175 = case shown="True" w44 {
          tunnel: w49 -> [_ w99]
          tunnel: w48 -> [_ w98]
          tunnel: [w96 w97] -> w40
          frame False {
            # "After the initial 2 seconds, do not reset \"Go now or wait?\""
            n176 = local read "Go now or wait?"() -> (w96:enum16{"Go Now", "Wait"})
          }
          frame True {
            n177 = case shown="\"No Target\"" w98 {
              tunnel: w99 -> [w102 _ w107]
              tunnel: [w103 enum16{"Go Now", "Wait"}."Go Now" w108] -> w97
              frame "Target Right", Default {
                # "IF on right and see\nright target, fire quickly.\nIf not, wait."
                n178 = Select(t=enum16{"Go Now", "Wait"}."Go Now", s=w102, f=enum16{"Go Now", "Wait"}."Wait") -> (s? t:f=w103:enum16{"Go Now", "Wait"})
              }
              frame "No Target" {
                # "If no target seen, fire ASAP"
              }
              frame "Target Left" {
                # "If on left and see\nleft target, fire quickly.\nIf not, wait."
                n179 = Select(t=enum16{"Go Now", "Wait"}."Wait", s=w107, f=enum16{"Go Now", "Wait"}."Go Now") -> (s? t:f=w108:enum16{"Go Now", "Wait"})
              }
            }
          }
        }
        "Go now or wait?" <- w40
        n180 = call <vilib>:"WPI_RobotDriveRefNum Registry Get.vi"("refnum name"="Left and Right Motors") -> ("RobotDriveDevRef"=w63:T20)  [unwired: 1 in, 9 out]
        n181 = call <vilib>:"WPI_SolenoidRefNum Registry Get.vi"("refnum name"="Shifter") -> ("error out"=w58:errorcluster, "SolenoidDevRef"=w57:T12)  [unwired: 9 in]
        n182 = call <vilib>:"WPI_SolenoidRefNum Registry Get.vi"("refnum name"="Shooter 3 & 4") -> ("error out"=w72:errorcluster, "SolenoidDevRef"=w76:T12)  [unwired: 9 in]
        n183 = call <vilib>:"WPI_SolenoidRefNum Registry Get.vi"("refnum name"="Lifter Arms") -> ("error out"=w54:errorcluster, "SolenoidDevRef"=w53:T12)  [unwired: 9 in]
        n184 = call-poly <vilib>:"WPI_SolenoidSet.vi"("error in (no error)"=w58, "Value"=WPI_SolenoidValue."Off", "SolenoidDevRef"=w57) -> ()  [unwired: 7 in, 2 out]
        n185 = call-poly <vilib>:"WPI_SolenoidSet.vi"("error in (no error)"=w72, "Value"=w65, "SolenoidDevRef"=w76) -> ()  [unwired: 7 in, 2 out]
        n186 = call <vilib>:"WPI_SolenoidRefNum Registry Get.vi"("refnum name"="Shooter Retract") -> ("error out"=w67:errorcluster, "SolenoidDevRef"=w66:T12)  [unwired: 9 in]
        n187 = call-poly <vilib>:"WPI_SolenoidSet.vi"("error in (no error)"=w54, "Value"=w52, "SolenoidDevRef"=w53) -> ()  [unwired: 7 in, 2 out]
        n188 = call-poly <vilib>:"WPI_SolenoidSet.vi"("error in (no error)"=w67, "Value"=w64, "SolenoidDevRef"=w66) -> ()  [unwired: 7 in, 2 out]
        n189 = call-poly <vilib>:"WPI_RobotDriveArcadeDrive.vi"("Y axis value"=w60, "X axis value"=0.0, "RobotDriveDevRef"=w63) -> ()  [unwired: 6 in, 3 out]
        n190 = call <vilib>:"WPI_SolenoidRefNum Registry Get.vi"("refnum name"="Shooter 2") -> ("error out"=w69:errorcluster, "SolenoidDevRef"=w77:T12)  [unwired: 9 in]
        n191 = call-poly <vilib>:"WPI_SolenoidSet.vi"("error in (no error)"=w69, "Value"=WPI_SolenoidValue."Off", "SolenoidDevRef"=w77) -> ()  [unwired: 7 in, 2 out]
        n192 = case shown="\"Go Now\", Default" w40 {
          tunnel: [w84 w91] -> w43
          tunnel: [w83 w90] -> w42
          tunnel: [w81 w88] -> w41
          tunnel: [w80 w87] -> w38
          frame "Go Now", Default {
            w80 = u32 1500 ("Drive Forward Time")
            n193 = Add(x=w80, y=u32 1700 ("Drive Forward Time")) -> (x+y=w81:u32)
            n194 = Add(x=w81, y=u32 500 ("Drive Forward Time")) -> (x+y=w83:u32)
            n195 = Add(x=w83, y=u32 1000 ("Open Arms Time")) -> (x+y=w84:u32)
          }
          frame "Wait" {
            w87 = u32 1500 ("Check Target Time")
            # "Add to make the bot wait."
            n196 = Add(x=w87, y=u32 1700 ("Drive Forward Time")) -> (x+y=w88:u32)
            n197 = Add(x=w88, y=u32 500 ("Drive Forward Time")) -> (x+y=w92:u32)
            n198 = Add(x=u32 4000, y=w92) -> (x+y=w90:u32)
            n199 = Add(x=w90, y=u32 1000 ("Open Arms Time")) -> (x+y=w91:u32)
          }
        }
        "Open Arms Time" <- w43
        "Drive Forward Time" <- w41
        "Stop Time" <- w42
        "Check Target Time" <- w38
        n200 = call <vilib>:"WPI_SolenoidRefNum Registry Get.vi"("refnum name"="Shooter 1") -> ("error out"=w74:errorcluster, "SolenoidDevRef"=w75:T12)  [unwired: 9 in]
        n201 = call-poly <vilib>:"WPI_SolenoidSet.vi"("error in (no error)"=w74, "Value"=w65, "SolenoidDevRef"=w75) -> ()  [unwired: 7 in, 2 out]
      }
    }
  }
  n202 = disable-structure shown="Enabled" {
    frame Disabled {
      w325 = "RobotDrive Motors" ("Name")
      # "This is some simple sample code to drive your robot curving one direction and then the other."
      # "stand still"
      # "turn left for 0.5 second"
      # "turn right for 1 second"
      n203 = call <vilib>:"WPI_RobotDriveRefNum Registry Get.vi"("refnum name"="Left and Right Motors") -> ("RobotDriveDevRef"=w329:T20)  [unwired: 1 in, 9 out]
      n204 = call-poly <vilib>:"WPI_RobotDriveArcadeDrive.vi"("Y axis value"=0.5 ("X axis value"), "X axis value"=0.25, "RobotDriveDevRef"=w329) -> ("Motor Values"=w328:dbl[], "RobotDriveDevRef"=w336:T20)  [unwired: 1 in, 6 out]
      n205 = call <vilib>:"SD Write Numeric Array.vi"("Numeric Array"=w328, "Name"=w325) -> ()  [unwired: 8 in, 2 out]
      n206 = call <vilib>:"WPI_RobotDriveDelayAndUpdateSafety.vi"("Delay (s)"=1.0, "RobotDriveDevRef"=w336) -> ("RobotDriveDevRef 2"=w335:T20)  [unwired: 8 in, 1 out]
      n207 = call-poly <vilib>:"WPI_RobotDriveArcadeDrive.vi"("Y axis value"=0.25 ("X axis value"), "X axis value"=0.5, "RobotDriveDevRef"=w335) -> ("Motor Values"=w327:dbl[], "RobotDriveDevRef"=w334:T20)  [unwired: 1 in, 6 out]
      n208 = call <vilib>:"SD Write Numeric Array.vi"("Numeric Array"=w327, "Name"=w325) -> ()  [unwired: 8 in, 2 out]
      n209 = call <vilib>:"WPI_RobotDriveDelayAndUpdateSafety.vi"("Delay (s)"=0.5, "RobotDriveDevRef"=w334) -> ("RobotDriveDevRef 2"=w333:T20)  [unwired: 8 in, 1 out]
      n210 = call-poly <vilib>:"WPI_RobotDriveArcadeDrive.vi"("Y axis value"=0.0 ("X axis value"), "X axis value"=0.0, "RobotDriveDevRef"=w333) -> ("Motor Values"=w326:dbl[])  [unwired: 1 in, 7 out]
      n211 = call <vilib>:"SD Write Numeric Array.vi"("Numeric Array"=w326, "Name"=w325) -> ()  [unwired: 8 in, 2 out]
    }
    frame Enabled {
    }
  }
  n212 = disable-structure shown="Enabled" {
    frame Disabled {
      # "This sample code describes robot movements in an array. You can extend it to control other motors\non your robot. You can also use file I/O to move the data to a text file."
      n213 = call <vilib>:"WPI_RobotDriveRefNum Registry Get.vi"("refnum name"="Left and Right Motors") -> ("RobotDriveDevRef"=w344:T20)  [unwired: 1 in, 9 out]
      n214 = for {
        shift-right: [w350] -> _
        shift-left: w344 -> [w351]
        tunnel: "Array of robot movements" -> [w346] mode=indexing
        n215 = Unbundle By Name(w346) -> ("X Joystick Value"=w349:dbl, "Y Joystick Value"=w348:dbl, "Delay (sec)"=w347:dbl)  [unwired: 1 out]
        n216 = call-poly <vilib>:"WPI_RobotDriveArcadeDrive.vi"("Y axis value"=w348, "X axis value"=w349, "RobotDriveDevRef"=w351) -> ("Motor Values"=w353:dbl[], "RobotDriveDevRef"=w352:T20)  [unwired: 1 in, 6 out]
        n217 = call <vilib>:"SD Write Numeric Array.vi"("Numeric Array"=w353, "Name"="RobotDrive Motors") -> ()  [unwired: 8 in, 2 out]
        n218 = call <vilib>:"WPI_RobotDriveDelayAndUpdateSafety.vi"("Delay (s)"=w347, "RobotDriveDevRef"=w352) -> ("RobotDriveDevRef 2"=w350:T20)  [unwired: 8 in, 1 out]
        "Current Movement, for debugging" <- w346
      }
    }
    frame Enabled {
    }
  }
